vi "Adder_service.vi"() -> ()   [LabVIEW 2010]
panel:
  out "# elements in queue":i32
  out "error out":errorcluster
  in  "attributes":string[][](array[string])=[["add_numbers", "(x:number, y:number) -> number"]]
  in  "Service Name":string="Adder"
  in  "Network Manager IP Address or Hostname":string
  in  "timeout ms":i32=10000
  in  "Network Manager port":u16=1875
  # "function name"
  # "function signature"
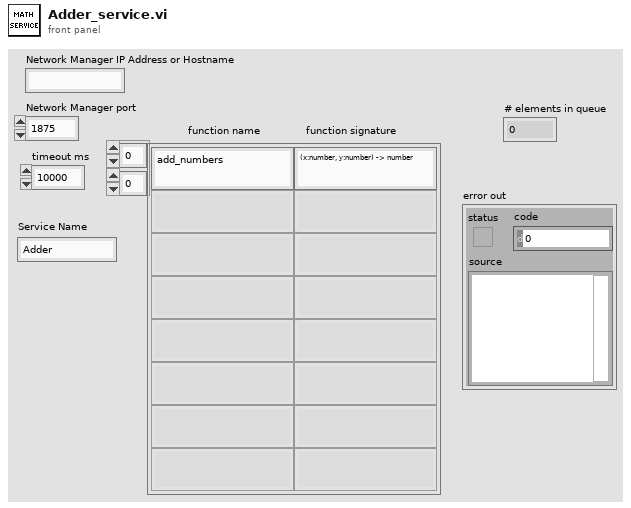
[diagram p1: front panel]
types:
  T1 = cluster{"type":u16, "name":string, "attributes":string[][]}
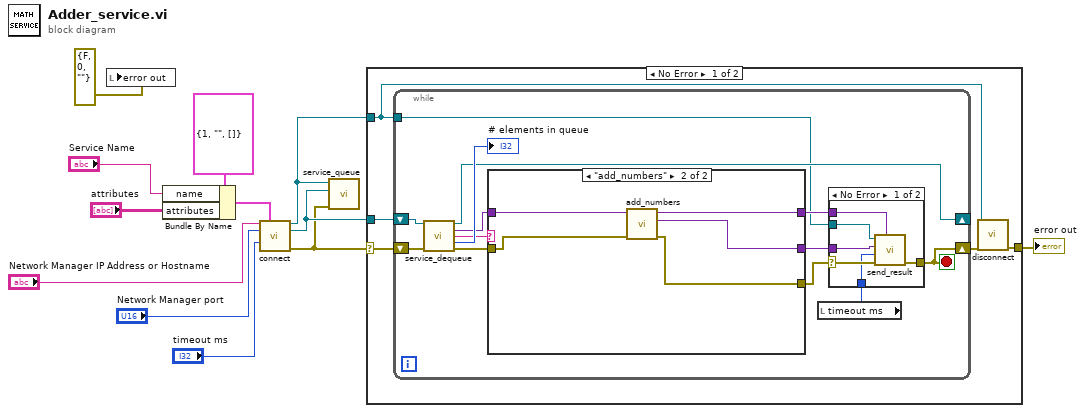
[diagram p0: block diagram]
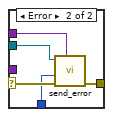
[diagram p2: hidden frame]
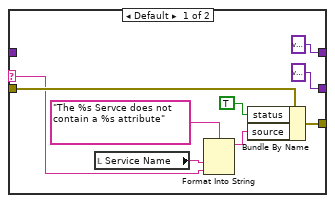
[diagram p3: hidden frame]
diagram:
  n1 = local write "error out"(errorcluster {"status"=FALSE, "code"=0, "source"=""} ("error out")) -> ()
  n2 = Bundle By Name(cluster=T1 {"type"=1, "name"="", "attributes"=[]} ("Identity"), "name"="Service Name", "attributes"="attributes") -> (w7:T1)
  n3 = call "connect.vi"("Network Manager IP Address or Hostname"="Network Manager IP Address or Hostname", "Identity"=w7, "Network Manager port"="Network Manager port", "timeout ms"="timeout ms") -> ("connection ID"=w3:refnum<k5>, "queue out"=w4:refnum<queue>, "error out"=w2:errorcluster)  [unwired: 9 in]
  n4 = call "service_queue.vi"("error in"=w2, "queue in"=w4, "connection ID"=w3) -> ()  [unwired: 9 in]
  n5 = case shown="No Error" w2 {
    selector: w2 -> [w13 w56]
    tunnel: w4 -> [w17 _]
    tunnel: w3 -> [w16 _]
    tunnel: [w14 w56] -> w1
    frame No Error {
      n6 = while {
        shift-right: [w29] -> w15
        shift-left: w13 -> [w27]
        shift-right: [w23] -> _
        shift-left: w17 -> [w28]
        tunnel: w16 -> [w18]
        stop <- w29 stop-if-true
        n7 = call "service_dequeue.vi"("queue"=w28, "error in"=w27) -> ("queue out"=w23:refnum<queue>, "JSON Tree Out Passthrough"=w22:variant, "function name"=w24:string, "# elements in queue"=→"# elements in queue":i32, "error out"=w26:errorcluster)  [unwired: 9 in]
        n8 = case shown="\"add_numbers\"" w24 {
          selector: w24 -> [w45 _]
          tunnel: w26 -> [w50 w55]
          tunnel: [w48 w53] -> w30
          tunnel: w22 -> [_ w54]
          tunnel: [variant ("JSON Tree Out Passthrough") w52] -> w21
          tunnel: [variant ("result") w51] -> w20
          frame Default {
            n9 = local read "Service Name"() -> (w46:string)
            n10 = Format Into String(format string="The %s Servce does not contain a %s attribute", w46, w45) -> (resulting string=w44:string)  [unwired: 2 in, 1 out]
            n11 = Bundle By Name(cluster=w50, "status"=TRUE, "source"=w44) -> (w48:errorcluster)
          }
          frame "add_numbers" {
            n12 = call "add_numbers.vi"("error in"=w55, "JSON Tree In (JSON Object)"=w54) -> ("error out"=w53:errorcluster, "result"=w51:variant, "JSON Tree Out Passthrough"=w52:variant)  [unwired: 7 in]
          }
        }
        n13 = local read "timeout ms"() -> (w19:i32)
        n14 = case shown="No Error" w30 {
          selector: w30 -> [w36 w41]
          tunnel: [w35 w40] -> w29
          tunnel: w18 -> [w34 w39]
          tunnel: w21 -> [w33 w37]
          tunnel: w20 -> [w32 _]
          tunnel: w19 -> [w31 w38]
          frame No Error {
            n15 = call "send_result.vi"("JSON Tree In (JSON Object)"=w33, "error in"=w36, "timeout ms"=w31, "result"=w32, "connection ID"=w34) -> ("error out"=w35:errorcluster)  [unwired: 3 in, 3 out]
          }
          frame Error {
            n16 = call "send_error.vi"("JSON Tree In (JSON Object)"=w37, "error in"=w41, "timeout ms"=w38, "connection ID"=w39) -> ("error out"=w40:errorcluster)  [unwired: 4 in, 3 out]
          }
        }
      }
      n17 = call "disconnect.vi"("error in (no error)"=w15, "connection ID"=w16) -> ("error out"=w14:errorcluster)  [unwired: 9 in]
    }
    frame Error {
    }
  }
  "error out" <- w1
